vi "hiddenLayerNode.vi"   [LabVIEW 2016]
uses:
  <vilib>/Analysis/Matrix/NI_Matrix.lvlib
  <vilib>/Analysis/Matrix/Numeric/Conversions/Matrix To Array - RM.vi
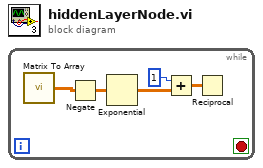
[diagram p0: block diagram]
diagram:
  n1 = while {
    stop <- _ stop-if-true
    n2 = call-poly <vilib>:"Matrix To Array.vi"() -> ("Real 2D Array"=w1:dbl[][])  [unwired: 1 in]
    n3 = Negate(x=w1) -> (-x=w3:dbl[][])
    n4 = Exponential(1:w3) -> (0:w4:dbl[][])
    n5 = Add(x=1, y=w4) -> (x+y=w2:dbl[][])
    n6 = Reciprocal(x=w2) -> ()  [unwired: 1 out]
  }
